vi "Cdeg Demo.vi"() -> ()   [LabVIEW 2012]
panel:
  out "Result":dbl[unit]
  in  "TempB":dbl[unit]
  in  "TempA":dbl[unit]=273.15
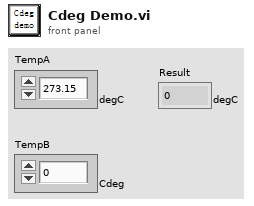
[diagram p1: front panel]
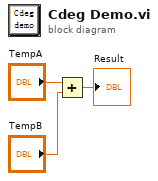
[diagram p0: block diagram]
diagram:
  n1 = Add(x="TempA", y="TempB") -> (x+y=→"Result":dbl[unit])
